vi "SimpleDataCollection.vi"() -> ()   [LabVIEW 2013]
uses:
  <vilib>/rvi/Emulation/niFpgaSctlEmulationGetInTimedLoop.vi
  <vilib>/rvi/Emulation/niFpgaEmulationReportErrorSimple.vi
  <vilib>/rvi/Emulation/niFpgaGetClockAttributes.vi
  <vilib>/rvi/eio/common/nirviEmuTemplateMethod_errors.vi
  <vilib>/rvi/Emulation/niFpgaCriticalErrorInLSC.vi
  <vilib>/eio/EIONode/EIONode.xnode
panel:
  in  "MCP":i16
  in  "PAC":i16
  out "Connector1/AI0":fxp<+/-,27,5>
  out "Count Register 11":u8
  out "Count Register 10":u8
  out "Count Register 9":u8
  out "Count Register 8":u8
  out "Count Register 7":u8
  out "Count Register 6":u8
  out "Count Register 5":u8
  out "Count Register 4":u8
  out "Count Register 3":u8
  out "Count Register 2":u8
  out "Count Register":u8
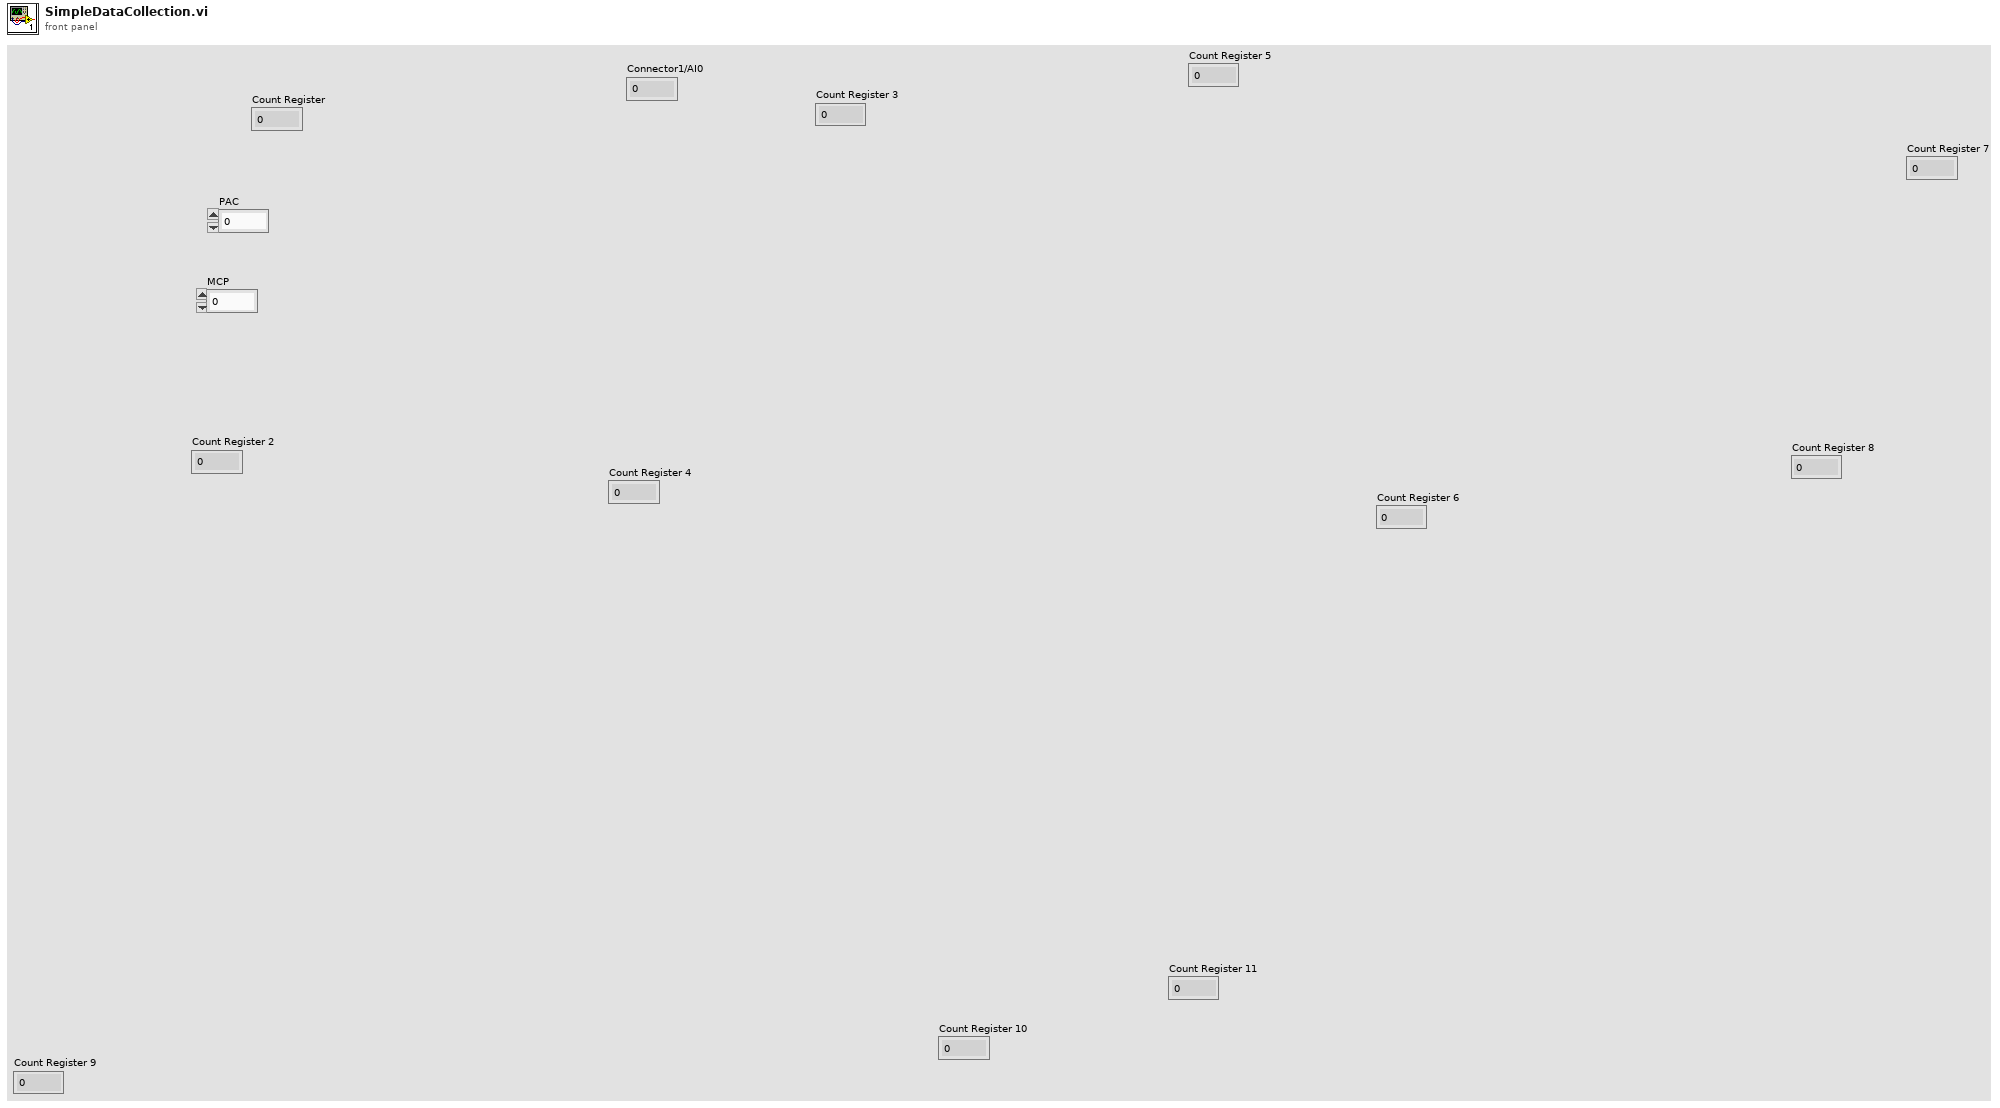
[diagram p1: front panel]
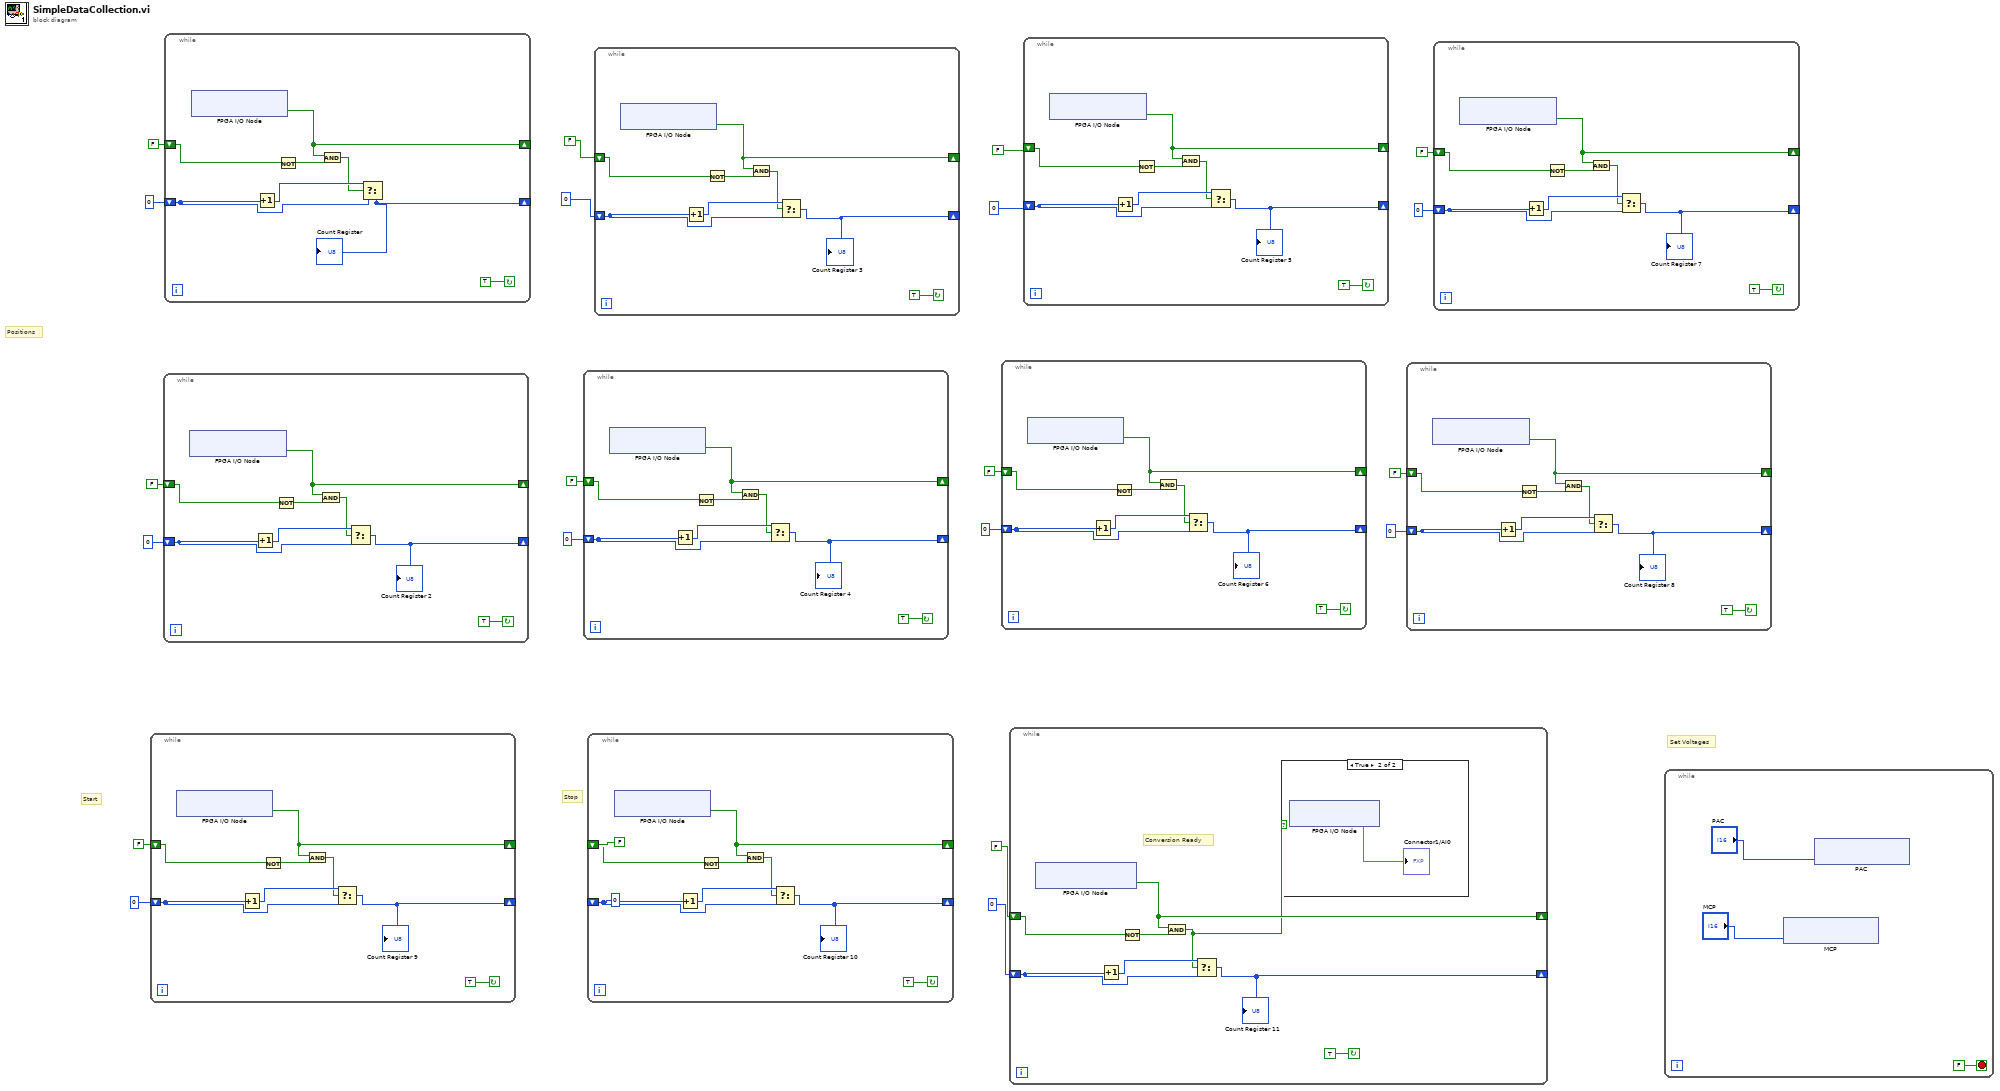
[diagram p0: block diagram]
diagram:
  # "Set Voltages"
  # "Stop"
  # "Start"
  # "Positions"
  n1 = while {
    shift-right: [w23] -> _
    shift-left: FALSE ("Connector0/DIO0") -> [w26]
    shift-right: [w27] -> _
    shift-left: u32 0 -> [w28]
    stop <- TRUE continue-if-true
    n2 = xnode "FPGA I/O Node"() -> ("Connector0/DIO8"=w23:bool)  [unwired: 1 in, 1 out]
    n3 = Increment(x=w28) -> (x+1=w29:u32)
    n4 = Not(x=w26) -> (.not. x?=w25:bool)
    n5 = And(x=w23, y=w25) -> (x .and. y?=w24:bool)
    n6 = Select(t=w29, s=w24, f=w28) -> (s? t:f=w27:u32)
    "Count Register 9" <- w27
  }
  n7 = while {
    shift-right: [w31] -> _
    shift-left: FALSE ("Connector0/DIO0") -> [w34]
    shift-right: [w35] -> _
    shift-left: u32 0 -> [w36]
    stop <- TRUE continue-if-true
    n8 = xnode "FPGA I/O Node"() -> ("Connector0/DIO1"=w31:bool)  [unwired: 1 in, 1 out]
    n9 = Increment(x=w36) -> (x+1=w37:u32)
    n10 = Not(x=w34) -> (.not. x?=w33:bool)
    n11 = And(x=w31, y=w33) -> (x .and. y?=w32:bool)
    n12 = Select(t=w37, s=w32, f=w36) -> (s? t:f=w35:u32)
    "Count Register 2" <- w35
  }
  n13 = while {
    shift-right: [w40] -> _
    shift-left: FALSE ("Connector0/DIO0") -> [w43]
    shift-right: [w39] -> _
    shift-left: u32 0 -> [w44]
    stop <- TRUE continue-if-true
    n14 = xnode "FPGA I/O Node"() -> ("Connector0/DIO0"=w40:bool)  [unwired: 1 in, 1 out]
    n15 = Increment(x=w44) -> (x+1=w45:u32)
    n16 = Not(x=w43) -> (.not. x?=w42:bool)
    n17 = And(x=w40, y=w42) -> (x .and. y?=w41:bool)
    n18 = Select(t=w45, s=w41, f=w44) -> (s? t:f=w39:u32)
    "Count Register" <- w39
  }
  n19 = while {
    shift-right: [w47] -> _
    shift-left: FALSE ("Connector0/DIO0") -> [w50]
    shift-right: [w51] -> _
    shift-left: u32 0 -> [w52]
    stop <- TRUE continue-if-true
    n20 = xnode "FPGA I/O Node"() -> ("Connector0/DIO3"=w47:bool)  [unwired: 1 in, 1 out]
    n21 = Increment(x=w52) -> (x+1=w53:u32)
    n22 = Not(x=w50) -> (.not. x?=w49:bool)
    n23 = And(x=w47, y=w49) -> (x .and. y?=w48:bool)
    n24 = Select(t=w53, s=w48, f=w52) -> (s? t:f=w51:u32)
    "Count Register 4" <- w51
  }
  n25 = while {
    shift-right: [w55] -> _
    shift-left: FALSE ("Connector0/DIO0") -> [w58]
    shift-right: [w59] -> _
    shift-left: u32 0 -> [w60]
    stop <- TRUE continue-if-true
    n26 = xnode "FPGA I/O Node"() -> ("Connector0/DIO9"=w55:bool)  [unwired: 1 in, 1 out]
    n27 = Increment(x=w60) -> (x+1=w61:u32)
    n28 = Not(x=w58) -> (.not. x?=w57:bool)
    n29 = And(x=w55, y=w57) -> (x .and. y?=w56:bool)
    n30 = Select(t=w61, s=w56, f=w60) -> (s? t:f=w59:u32)
    "Count Register 10" <- w59
  }
  n31 = while {
    shift-right: [w63] -> _
    shift-left: FALSE ("Connector0/DIO0") -> [w66]
    shift-right: [w67] -> _
    shift-left: u32 0 -> [w68]
    stop <- TRUE continue-if-true
    n32 = xnode "FPGA I/O Node"() -> ("Connector0/DIO2"=w63:bool)  [unwired: 1 in, 1 out]
    n33 = Increment(x=w68) -> (x+1=w69:u32)
    n34 = Not(x=w66) -> (.not. x?=w65:bool)
    n35 = And(x=w63, y=w65) -> (x .and. y?=w64:bool)
    n36 = Select(t=w69, s=w64, f=w68) -> (s? t:f=w67:u32)
    "Count Register 3" <- w67
  }
  n37 = while {
    shift-right: [w71] -> _
    shift-left: FALSE ("Connector0/DIO0") -> [w74]
    shift-right: [w75] -> _
    shift-left: u32 0 -> [w76]
    stop <- TRUE continue-if-true
    n38 = xnode "FPGA I/O Node"() -> ("Connector0/DIO5"=w71:bool)  [unwired: 1 in, 1 out]
    n39 = Increment(x=w76) -> (x+1=w77:u32)
    n40 = Not(x=w74) -> (.not. x?=w73:bool)
    n41 = And(x=w71, y=w73) -> (x .and. y?=w72:bool)
    n42 = Select(t=w77, s=w72, f=w76) -> (s? t:f=w75:u32)
    "Count Register 6" <- w75
  }
  n43 = while {
    shift-right: [w80] -> _
    shift-left: FALSE ("Connector0/DIO0") -> [w82]
    shift-right: [w83] -> _
    shift-left: u32 0 -> [w84]
    stop <- TRUE continue-if-true
    # "Conversion Ready"
    n44 = xnode "FPGA I/O Node"() -> ("Connector0/DIO10"=w80:bool)  [unwired: 1 in, 1 out]
    n45 = Increment(x=w84) -> (x+1=w85:u32)
    n46 = Not(x=w82) -> (.not. x?=w81:bool)
    n47 = And(x=w80, y=w81) -> (x .and. y?=w79:bool)
    n48 = Select(t=w85, s=w79, f=w84) -> (s? t:f=w83:u32)
    "Count Register 11" <- w83
    n49 = case shown="True" w79 {
      frame False {
      }
      frame True {
        n50 = xnode "FPGA I/O Node"() -> ("Connector1/AI0"=→"Connector1/AI0":fxp<+/-,27,5>)  [unwired: 1 in, 1 out]
      }
    }
  }
  n51 = while {
    shift-right: [w88] -> _
    shift-left: FALSE ("Connector0/DIO0") -> [w91]
    shift-right: [w92] -> _
    shift-left: u32 0 -> [w93]
    stop <- TRUE continue-if-true
    n52 = xnode "FPGA I/O Node"() -> ("Connector0/DIO4"=w88:bool)  [unwired: 1 in, 1 out]
    n53 = Increment(x=w93) -> (x+1=w94:u32)
    n54 = Not(x=w91) -> (.not. x?=w90:bool)
    n55 = And(x=w88, y=w90) -> (x .and. y?=w89:bool)
    n56 = Select(t=w94, s=w89, f=w93) -> (s? t:f=w92:u32)
    "Count Register 5" <- w92
  }
  n57 = while {
    shift-right: [w96] -> _
    shift-left: FALSE ("Connector0/DIO0") -> [w99]
    shift-right: [w100] -> _
    shift-left: u32 0 -> [w101]
    stop <- TRUE continue-if-true
    n58 = xnode "FPGA I/O Node"() -> ("Connector0/DIO7"=w96:bool)  [unwired: 1 in, 1 out]
    n59 = Increment(x=w101) -> (x+1=w102:u32)
    n60 = Not(x=w99) -> (.not. x?=w98:bool)
    n61 = And(x=w96, y=w98) -> (x .and. y?=w97:bool)
    n62 = Select(t=w102, s=w97, f=w101) -> (s? t:f=w100:u32)
    "Count Register 8" <- w100
  }
  n63 = while {
    shift-right: [w104] -> _
    shift-left: FALSE ("Connector0/DIO0") -> [w107]
    shift-right: [w108] -> _
    shift-left: u32 0 -> [w109]
    stop <- TRUE continue-if-true
    n64 = xnode "FPGA I/O Node"() -> ("Connector0/DIO6"=w104:bool)  [unwired: 1 in, 1 out]
    n65 = Increment(x=w109) -> (x+1=w110:u32)
    n66 = Not(x=w107) -> (.not. x?=w106:bool)
    n67 = And(x=w104, y=w106) -> (x .and. y?=w105:bool)
    n68 = Select(t=w110, s=w105, f=w109) -> (s? t:f=w108:u32)
    "Count Register 7" <- w108
  }
  n69 = while {
    stop <- FALSE stop-if-true
    n70 = xnode "MCP"("Connector1/AO1"="MCP") -> ()  [unwired: 1 in, 1 out]
    n71 = xnode "PAC"("Connector1/AO0"="PAC") -> ()  [unwired: 1 in, 1 out]
  }
